vi "SetWindowsClock.vi"(8 "error in (no error)":errorcluster, 9 "time stamp":timestamp, 10 "SyncWinClk":bool, 11 "SyncPluginBase in":refnum<class "SyncPluginBase.lvclass">) -> (0 "error out":errorcluster, 3 "SyncPluginBase out":refnum<class "SyncPluginBase.lvclass">)   [LabVIEW 2014, in "SyncPlugins.lvlib" / "SyncPluginBase.lvclass"]
uses:
  SyncPluginBase.lvclass
  kernel32.dll
panel:
  out "WindowsTime":T1
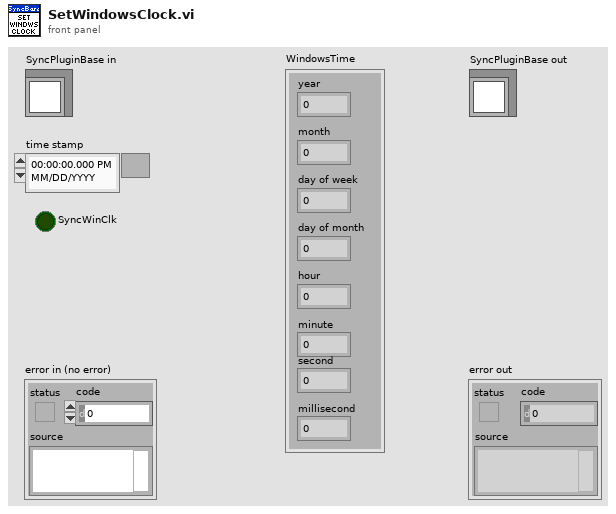
[diagram p1: front panel]
types:
  T1 = cluster{"year":i16, "month":i16, "day of week":i16, "day of month":i16, "hour":i16, "minute":i16, "second":i16, "millisecond":i16}
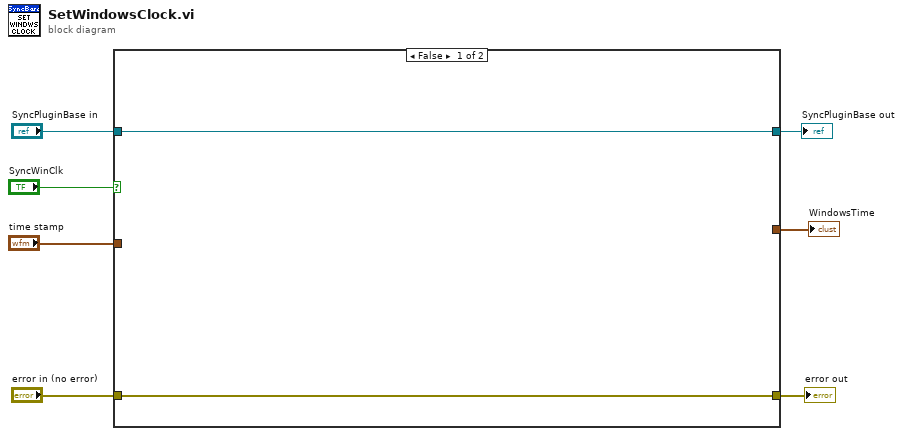
[diagram p0: block diagram]
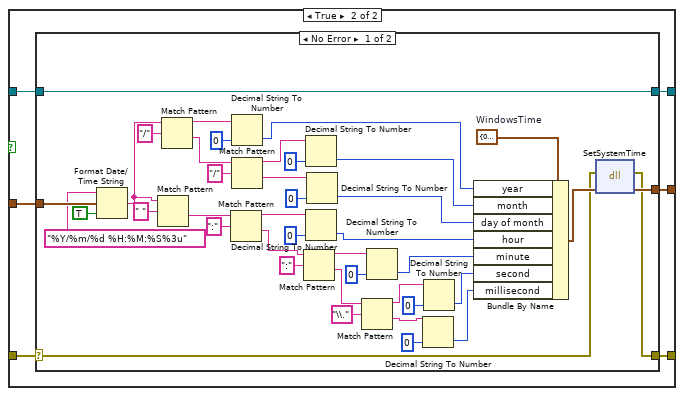
[diagram p2: hidden frame]
diagram:
  n1 = case shown="False" "SyncWinClk" {
    tunnel: "error in (no error)" -> [w8 w15]
    tunnel: [w8 w14] -> w6
    tunnel: "SyncPluginBase in" -> [w9 w13]
    tunnel: [w9 w12] -> w4
    tunnel: "time stamp" -> [_ w11]
    tunnel: [_ w10] -> w2
    frame False {
    }
    frame True {
      n2 = case shown="No Error" w15 {
        selector: w15 -> [w18 w58]
        tunnel: [w17 w58] -> w14
        tunnel: [w56 w57] -> w12
        tunnel: w13 -> [w56 w57]
        tunnel: w11 -> [w41 _]
        tunnel: [w53 _] -> w10
        frame No Error {
          w55 = T1 {"year"=0, "month"=0, "day of week"=0, "day of month"=0, "hour"=0, "minute"=0, "second"=0, "millisecond"=0}  # WindowsTime
          n3 = Format Date/Time String(time format string (%c)="%Y/%m/%d %H:%M:%S%3u", seconds (now)=w41, UTC format=TRUE) -> (date/time string=w36:string)
          n4 = Match Pattern(string=w36, regular expression=" ") -> (after substring=w35:string)  [unwired: 1 in, 3 out]
          n5 = Match Pattern(string=w36, regular expression="/") -> (before substring=w50:string, after substring=w48:string)  [unwired: 1 in, 2 out]
          n6 = Match Pattern(string=w35, regular expression=":") -> (before substring=w31:string, after substring=w29:string)  [unwired: 1 in, 2 out]
          n7 = Decimal String To Number(string=w50, default (0L)=i16 0 ("default (0 I32)")) -> (number=w43:i16)  [unwired: 1 in, 1 out]
          n8 = Match Pattern(string=w48, regular expression="/") -> (before substring=w46:string, after substring=w44:string)  [unwired: 1 in, 2 out]
          n9 = Match Pattern(string=w29, regular expression=":") -> (before substring=w27:string, after substring=w24:string)  [unwired: 1 in, 2 out]
          n10 = Decimal String To Number(string=w46, default (0L)=i16 0 ("default (0 I32)")) -> (number=w39:i16)  [unwired: 1 in, 1 out]
          n11 = Decimal String To Number(string=w31, default (0L)=i16 0 ("default (0 I32)")) -> (number=w30:i16)  [unwired: 1 in, 1 out]
          n12 = Decimal String To Number(string=w44, default (0L)=i16 0 ("default (0 I32)")) -> (number=w38:i16)  [unwired: 1 in, 1 out]
          n13 = Match Pattern(string=w24, regular expression="\\.") -> (before substring=w22:string, after substring=w19:string)  [unwired: 1 in, 2 out]
          n14 = Decimal String To Number(string=w27, default (0L)=i16 0 ("default (0 I32)")) -> (number=w26:i16)  [unwired: 1 in, 1 out]
          n15 = Decimal String To Number(string=w19, default (0L)=i16 0 ("default (0 I32)")) -> (number=w16:i16)  [unwired: 1 in, 1 out]
          n16 = Decimal String To Number(string=w22, default (0L)=i16 0 ("default (0 I32)")) -> (number=w21:i16)  [unwired: 1 in, 1 out]
          n17 = Bundle By Name(cluster=w55, "year"=w43, "month"=w39, "day of month"=w38, "hour"=w30, "minute"=w26, "second"=w21, "millisecond"=w16) -> (w54:T1)
          n18 = dll-call lib="kernel32.dll" fn="SetSystemTime"(error in=w18, "time"=w54) -> (error out=w17:errorcluster, "time"=w53:T1)  [unwired: 3 in, 1 out]
        }
        frame Error {
        }
      }
    }
  }
  "error out" <- w6
  "SyncPluginBase out" <- w4
  "WindowsTime" <- w2
